vi "DotNETCam_TemplateMethod.vi"(8 "ErrorIn":errorcluster, 10 "CmdData":variant, 11 "DotNETCamIn":refnum<class>) -> (0 "ErrorOut":errorcluster, 2 "ReplyData":variant, 3 "DotNETCamOut":refnum<class>, 4 "Exit":bool)   [LabVIEW 2021, in "DotNETCam.lvclass"]
uses:
  DotNETCam.lvclass
  DotNETCam_MsgCtrl.ctl
  DotNETCam.lvclass/DotNETCam.ctl
  C:/Localdata/Projects/TriekselSoft/TriekselsoftApplicationFramework/Source/.Externals/Library_YAF/YAFTAF/YAFTAF.lvclass
  C:/Localdata/Projects/TriekselSoft/TriekselsoftApplicationFramework/Source/.Externals/Library_YAF/YActor/YActor.lvclass
  C:/Localdata/Projects/TriekselSoft/TriekselsoftApplicationFramework/Source/.Externals/Interface_UserInterface_IFrontPanel/IFrontPanel/IFrontPanel.lvclass
  C:/Localdata/Projects/TriekselSoft/TriekselsoftApplicationFramework/Source/IInterface/IInterface.lvclass
  C:/Localdata/Projects/TriekselSoft/TriekselsoftApplicationFramework/Source/.Externals/Interface_Object_ICreateDestroy/ICreateDestroy/ICreateDestroy.lvclass
  C:/Localdata/Projects/TriekselSoft/TriekselsoftApplicationFramework/Source/.Externals/Interface_Object_IPersistentData/IPersistentData/IPersistentData.lvclass
  C:/Localdata/Projects/TriekselSoft/TriekselsoftApplicationFramework/Source/.Externals/Interface_TAF_ITAFObject/ITAFObject/ITAFObject.lvclass
  C:/Localdata/Projects/TriekselSoft/TriekselsoftApplicationFramework/Source/YAFTAFObjects/DotNETCam/DotNETCam.lvclass
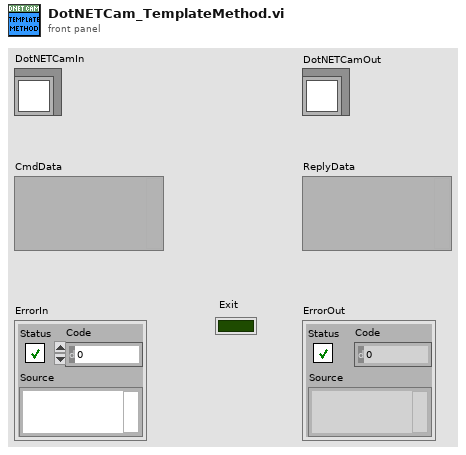
[diagram p1: front panel]
types:
  T1 = typedef "DotNETCam.lvclass/DotNETCam_MsgCtrl.ctl" = cluster{"TemplateCommand":cluster{"DummyIn":dbl, "DummyOut":dbl}}
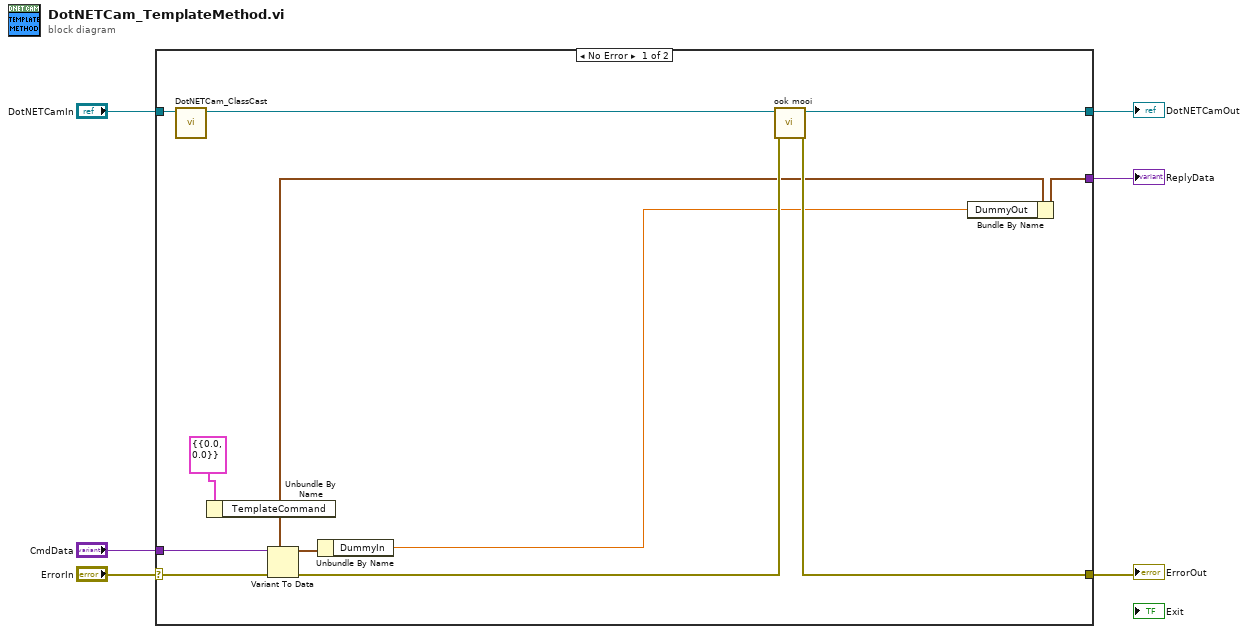
[diagram p0: block diagram]
diagram:
  n1 = case shown="No Error" "ErrorIn" {
    selector: "ErrorIn" -> [w18 w21]
    tunnel: [w16 w21] -> w5
    tunnel: [w8 w20] -> w3
    tunnel: "CmdData" -> [w14 w20]
    tunnel: "DotNETCamIn" -> [w15 w19]
    tunnel: [w7 w19] -> w1
    frame No Error {
      n2 = call "DotNETCam_ClassCast.vi"("DotNETCamIn"=w15) -> ("DotNETCamOut"=w11:refnum<class "DotNETCam.lvclass">)  [unwired: 10 in]
      n3 = Unbundle By Name(T1 {"TemplateCommand"={"DummyIn"=0.0, "DummyOut"=0.0}} ("MsgData")) -> ("TemplateCommand"=w10:cluster{"DummyIn":dbl, "DummyOut":dbl})
      n4 = Variant To Data(error in=w18, type=w10, Variant=w14) -> (data=w12:cluster{"DummyIn":dbl, "DummyOut":dbl}, error out=w17:errorcluster)
      n5 = Unbundle By Name(w12) -> ("DummyIn"=w9:dbl)
      n6 = call-dynamic "ook mooi.vi"("error in (no error)"=w17, "DotNETCam in"=w11) -> ("error out"=w16:errorcluster, "DotNETCam out"=w7:refnum<class "DotNETCam.lvclass">)  [unwired: 7 in, 1 out]
      n7 = Bundle By Name(cluster=w10, "DummyOut"=w9) -> (w8:cluster{"DummyIn":dbl, "DummyOut":dbl})
    }
    frame Error {
    }
  }
  "ErrorOut" <- w5
  "DotNETCamOut" <- w1
  "ReplyData" <- w3
